vi "Datalogger.vi"   [LabVIEW 2015]
uses:
  DAQ/Controls/Channel Configuration.ctl
  CAN Communication/Oil/Typedefs/Session Handle.ctl
  CAN Communication/Oil/Oil.lvclass
  Common/Buffers/Snapshot/Typedefs/Session Handle.ctl
  Common/Buffers/Snapshot/Snapshot.lvclass
  Common/Circular Error Log/Typedefs/Session Handle.ctl
  Common/Circular Error Log/Circular Error Log.lvclass
  Common/State Machine/State Machine.lvlib
panel:
  # "Datalogger"
types:
  T1 = typedef "Channel Configuration.ctl" = cluster{"Index":u16, "Name":string, "Units":string, "Gain":dbl, "Offset":dbl, "Source":string}
  T2 = typedef "Oil.lvclass/Session Handle.ctl" = refnum<data-value>
  T3 = typedef "Snapshot.lvclass/Session Handle.ctl" = refnum<data-value>
  T4 = typedef "Circular Error Log.lvclass/Session Handle.ctl" = refnum<data-value>
  T5 = cluster{"State":refnum<queue>, "Channels":T1[], "Oil":T2, "Snapshot":T3, "Log Reference":refnum<file>, "LogData":refnum<queue>, "Error":T4, "Log Folder":path}
  T6 = cluster{"Averaged Values":dbl[], "seconds since 1Jan1904":timestamp}
  T7 = enum16{"open", "replace", "create", "open or create", "replace or create", "replace or create with confirmation"}
  T8 = cluster{"Test Name":string, "Test Start":timestamp}
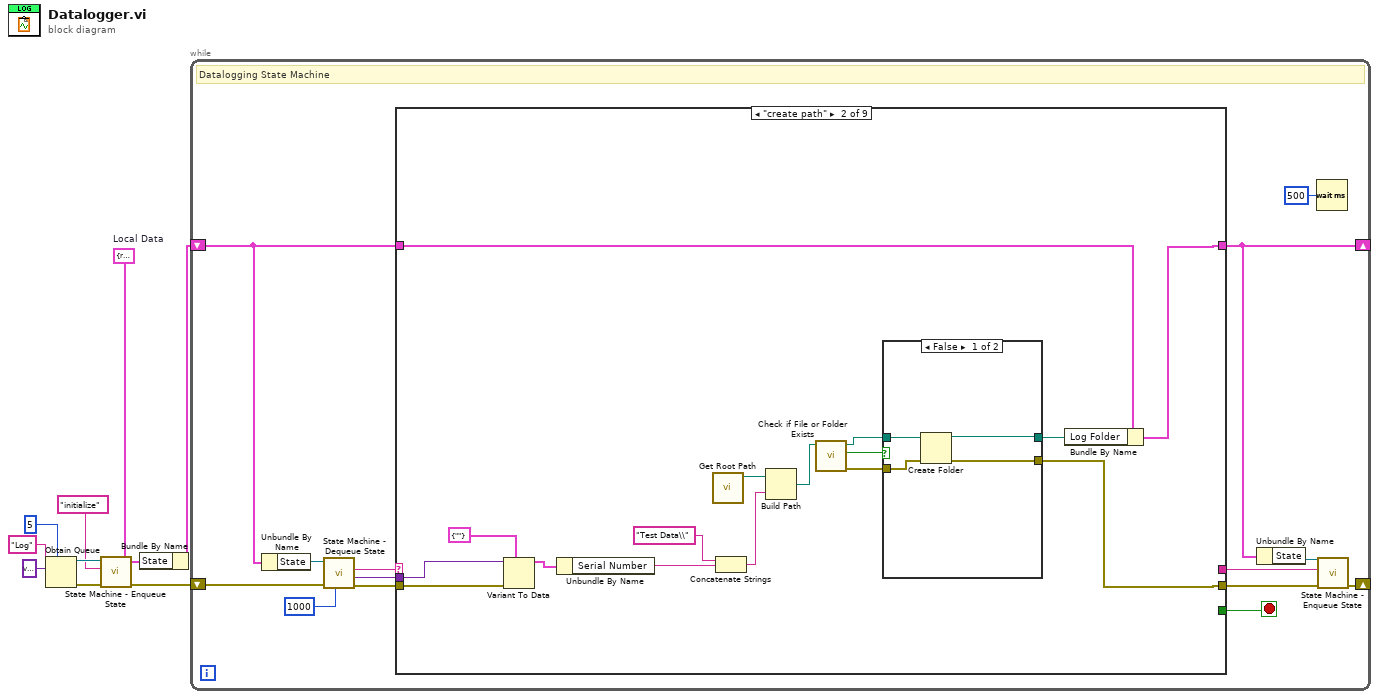
[diagram p0: block diagram]
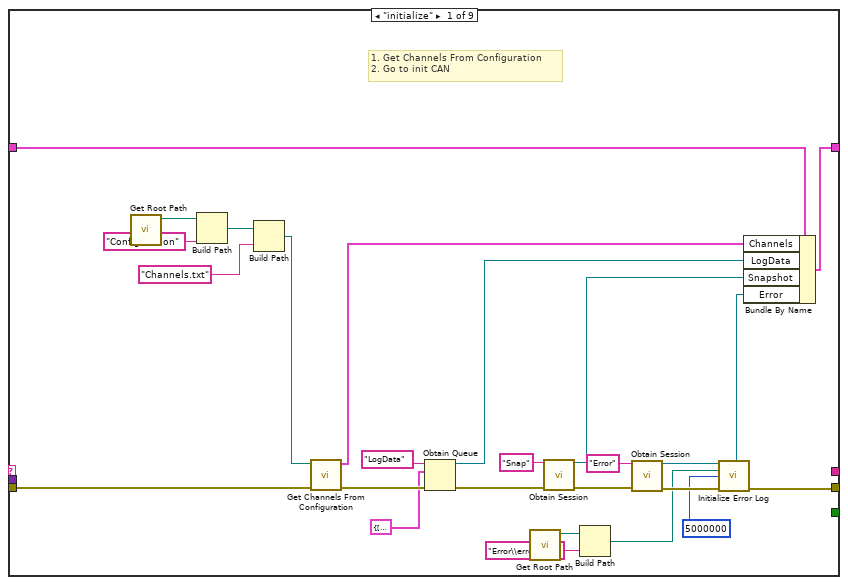
[diagram p2: hidden frame]
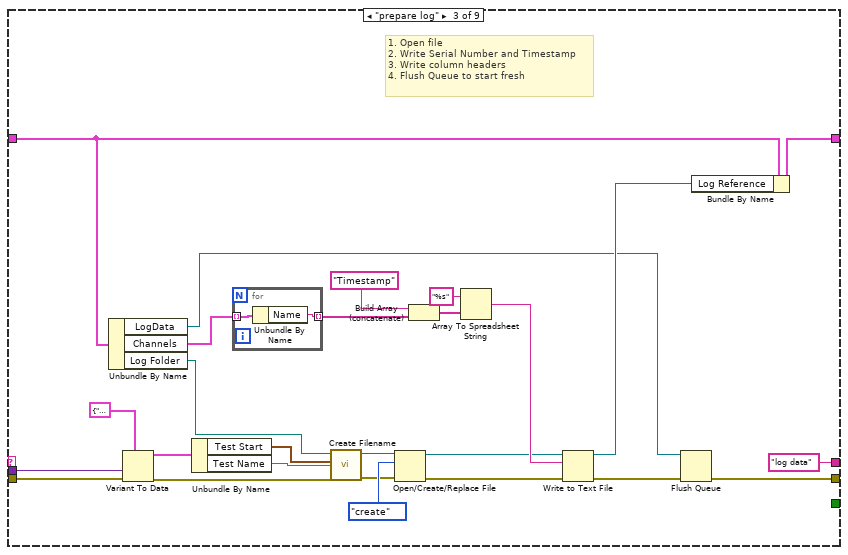
[diagram p4: hidden frame]
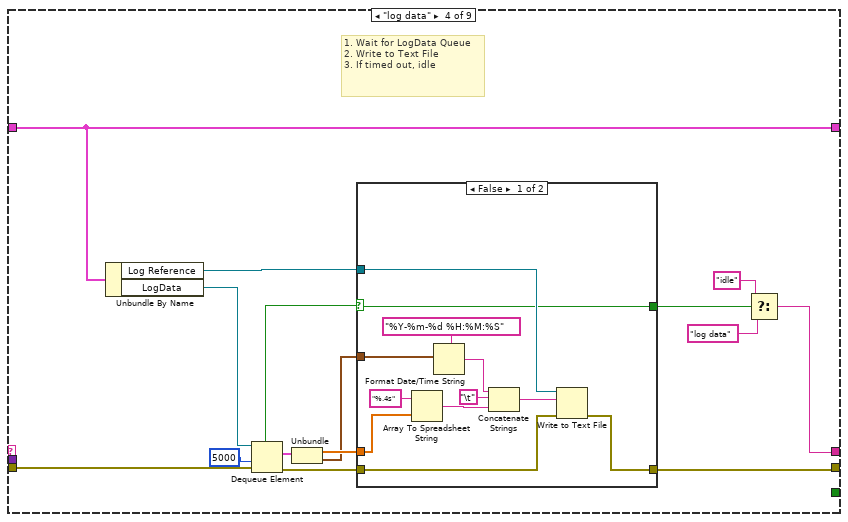
[diagram p5: hidden frame]
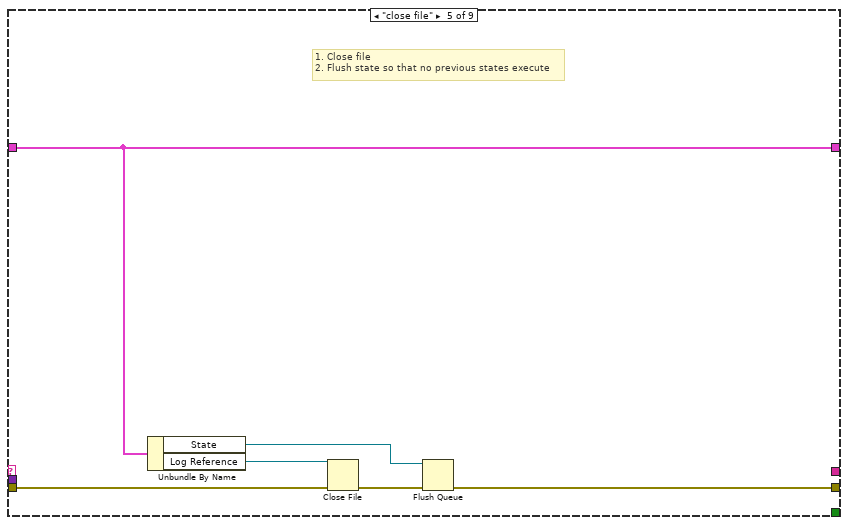
[diagram p7: hidden frame]
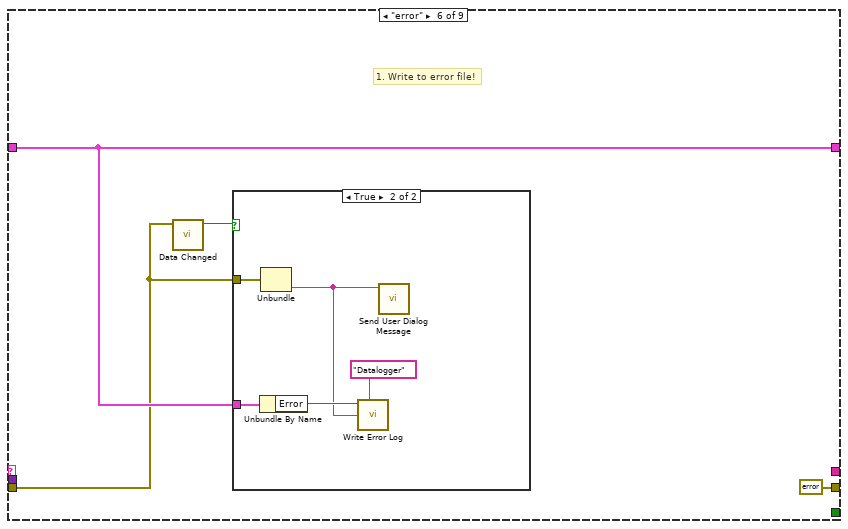
[diagram p8: hidden frame]
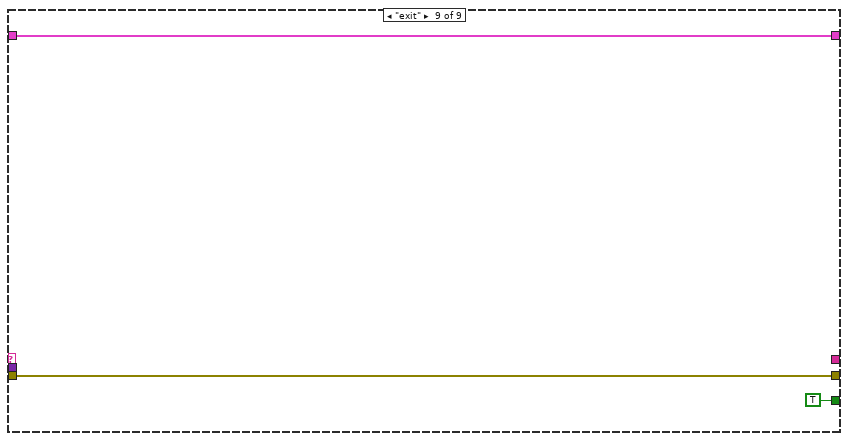
[diagram p12: hidden frame]
diagram:
  w3 = T5 {"State"=refnum, "Channels"=[], "Oil"=refnum, "Snapshot"=refnum, "Log Reference"=refnum, "LogData"=refnum, "Error"=refnum, "Log Folder"=path ""}  # Local Data
  n1 = Obtain Queue(max queue size (-1, unlimited)=5, name (unnamed)="Log", element data type=variant) -> (queue out=w6:refnum<queue>, error out=w7:errorcluster)  [unwired: 2 in, 1 out]
  n2 = call "State Machine - Enqueue State.vi"("error in (no error)"=w7, "State"="initialize", "Queue In"=w6) -> ("error out"=w4:errorcluster, "Queue Out"=w2:refnum<queue>)  [unwired: 7 in]
  n3 = Bundle By Name(cluster=w3, "State"=w2) -> (w1:T5)
  n4 = while "Main State Machine" {
    shift-right: [w21] -> _
    shift-left: w4 -> [w24]
    shift-right: [w12] -> _
    shift-left: w1 -> [w15]
    stop <- w17 stop-if-true
    # "Datalogging State Machine"
    n5 = Unbundle By Name(w15) -> ("State"=w14:refnum<queue>)
    n6 = call "State Machine - Dequeue State.vi"("Timeout"=1000, "error in (no error)"=w24, "Queue In"=w14) -> ("error out"=w23:errorcluster, "Data"=w11:variant, "State"=w22:string)  [unwired: 4 in, 2 out]
    n7 = case shown="\"create path\"" w22 {
      tunnel: w23 -> [w47 w65 w98 w110 w133 w137 w146 w148 w151]
      tunnel: [w30 w51 w78 w105 w130 errorcluster {"status"=FALSE, "code"=0, "source"=""} ("error out") w146 w148 w151] -> w20
      tunnel: [_ _ "log data" ("State") w113 _ _ _ _ _] -> w19
      tunnel: [_ _ _ _ _ _ _ _ TRUE] -> w17
      tunnel: w15 -> [w45 w54 w90 w115 w135 w138 w145 w147 w149]
      tunnel: [w44 w53 w89 w115 w135 w138 w145 w147 w149] -> w12
      tunnel: w11 -> [_ w64 w97 _ _ _ _ _ _]
      frame "initialize" {
        # "1. Get Channels From Configuration\n2. Go to init CAN"
        n8 = call "Get Root Path.vi"() -> ("Root Path"=w28:path)  [unwired: 11 in]
        n9 = Build Path(base path=w28, name or relative path="Configuration") -> (appended path=w49:path)
        n10 = Build Path(base path=w49, name or relative path="Channels.txt") -> (appended path=w46:path)
        n11 = call "Get Channels From Configuration.vi"("error in (no error)"=w47, "Path"=w46) -> ("error out"=w42:errorcluster, "Channels"=w43:T1[])  [unwired: 8 in]
        n12 = Obtain Queue(name (unnamed)="LogData", element data type=T6 {"Averaged Values"=[], "seconds since 1Jan1904"=timestamp(0 s since 1904-01-01)} ("output cluster"), error in (no error)=w42) -> (queue out=w40:refnum<queue>, error out=w39:errorcluster)  [unwired: 2 in, 1 out]
        n13 = call "Get Root Path.vi"() -> ("Root Path"=w27:path)  [unwired: 11 in]
        n14 = call "Obtain Session.vi"("Session  Name ()"="Snap", "error in (no error)"=w39) -> ("Session Handle"=w37:T3, "error out"=w31:errorcluster)  [unwired: 12 in]
        n15 = Build Path(base path=w27, name or relative path="Error\\error.txt") -> (appended path=w25:path)
        n16 = call "Obtain Session.vi"("Session  Name ()"="Error", "error in (no error)"=w31) -> ("Session Handle"=w33:T4, "error out"=w34:errorcluster)  [unwired: 12 in]
        n17 = call "Initialize Error Log.vi"("Session Handle in"=w33, "Error Path"=w25, "Max File Size"=i64 5000000, "error in (no error)"=w34) -> ("Session Handle out"=w29:T4, "error out"=w30:errorcluster)  [unwired: 10 in]
        n18 = Bundle By Name(cluster=w45, "Channels"=w43, "LogData"=w40, "Snapshot"=w37, "Error"=w29) -> (w44:T5)
      }
      frame "create path" {
        n19 = Variant To Data(error in=w65, type=cluster{"Serial Number":string} {"Serial Number"=""}, Variant=w64) -> (data=w63:cluster{"Serial Number":string})  [unwired: 1 out]
        n20 = Unbundle By Name(w63) -> ("Serial Number"=w61:string)
        n21 = call "Get Root Path.vi"() -> ("Root Path"=w62:path)  [unwired: 11 in]
        n22 = Concatenate Strings("Test Data\\" ("string"), w61) -> (w59:string)
        n23 = Build Path(base path=w62, name or relative path=w59) -> (appended path=w58:path)
        n24 = call <vilib>:"Check if File or Folder Exists.vi"("path"=w58) -> ("error out"=w55:errorcluster, "file or folder exists?"=w57:bool, "dup path"=w56:path)  [unwired: 8 in]
        n25 = case shown="False" w57 {
          tunnel: [w68 w72] -> w52
          tunnel: w56 -> [w70 w72]
          tunnel: w55 -> [w69 w71]
          tunnel: [w67 w71] -> w51
          frame False {
            n26 = Create Folder(path (use dialog)=w70, error in=w69) -> (created path=w68:path, error out=w67:errorcluster)  [unwired: 1 in, 1 out]
          }
          frame True {
          }
        }
        n27 = Bundle By Name(cluster=w54, "Log Folder"=w52) -> (w53:T5)
      }
      frame "prepare log" {
        # "1. Open file\n2. Write Serial Number and Timestamp\n3. Write column headers\n4. Flush Queue to start fresh"
        n28 = Unbundle By Name(w90) -> ("LogData"=w79:refnum<queue>, "Channels"=w88:T1[], "Log Folder"=w73:path)
        n29 = Variant To Data(error in=w98, type=T8 {"Test Name"="", "Test Start"=timestamp(0 s since 1904-01-01)}, Variant=w97) -> (data=w95:T8, error out=w75:errorcluster)
        n30 = Unbundle By Name(w95) -> ("Test Start"=w94:timestamp, "Test Name"=w93:string)
        n31 = for {
          tunnel: w88 -> [w100] mode=indexing
          tunnel: [w99] -> w87 mode=indexing
          n32 = Unbundle By Name(w100) -> ("Name"=w99:string)
        }
        n33 = call "Create Filename.vi"("error in (no error)"=w75, "Test Name"=w93, "Test Start"=w94, "Data Folder"=w73) -> ("error out"=w74:errorcluster, "appended path out"=w92:path)  [unwired: 6 in]
        n34 = Open/Create/Replace File(file path (use dialog)=w92, error in=w74, operation (0:open)=T7."create") -> (refnum out=w81:refnum<file>, error out=w83:errorcluster)  [unwired: 3 in, 1 out]
        n35 = Build Array (concatenate)("Timestamp" ("Name"), w87) -> (w85:string[])
        n36 = Array To Spreadsheet String(array=w85, 3:"%s" ("format string")) -> (spreadsheet string=w82:string)  [unwired: 1 in]
        n37 = Write to Text File(file (use dialog)=w81, text=w82, error in=w83) -> (refnum out=w80:refnum<file>, error out=w77:errorcluster)  [unwired: 1 in, 1 out]
        n38 = Flush Queue(queue=w79, error in (no error)=w77) -> (error out=w78:errorcluster)  [unwired: 2 out]
        n39 = Bundle By Name(cluster=w90, "Log Reference"=w80) -> (w89:T5)
      }
      frame "log data" {
        # "1. Wait for LogData Queue\n2. Write to Text File\n3. If timed out, idle"
        n40 = Unbundle By Name(w115) -> ("Log Reference"=w106:refnum<file>, "LogData"=w114:refnum<queue>)
        n41 = Dequeue Element(queue=w114, timeout in ms (-1)=5000, error in (no error)=w110) -> (element=w102:T6, timed out?=w107:bool, error out=w108:errorcluster)  [unwired: 1 out]
        n42 = Unbundle(w102) -> ("Averaged Values"=w103:dbl[], "seconds since 1Jan1904"=w101:timestamp)
        n43 = case shown="False" w107 {
          selector: w107 -> [w122 w128]
          tunnel: w108 -> [w125 w129]
          tunnel: w103 -> [w127 _]
          tunnel: w106 -> [w124 _]
          tunnel: [w123 w129] -> w105
          tunnel: [w122 w128] -> w104
          tunnel: w101 -> [w116 _]
          frame False {
            n44 = Array To Spreadsheet String(array=w127, 3:"%.4s" ("format string")) -> (spreadsheet string=w118:string)  [unwired: 1 in]
            n45 = Format Date/Time String(time format string (%c)="%Y-%m-%d %H:%M:%S", seconds (now)=w116) -> (date/time string=w120:string)  [unwired: 1 in]
            n46 = Concatenate Strings(w120, "\t", w118) -> (w117:string)
            n47 = Write to Text File(file (use dialog)=w124, text=w117, error in=w125) -> (error out=w123:errorcluster)  [unwired: 1 in, 2 out]
          }
          frame True {
          }
        }
        n48 = Select(t="idle" ("State"), s=w104, f="log data" ("State")) -> (s? t:f=w113:string)
      }
      frame "close file" {
        # "1. Close file\n2. Flush state so that no previous states execute"
        n49 = Unbundle By Name(w135) -> ("State"=w131:refnum<queue>, "Log Reference"=w134:refnum<file>)
        n50 = Close File(refnum=w134, error in=w133) -> (error out=w132:errorcluster)  [unwired: 1 out]
        n51 = Flush Queue(queue=w131, error in (no error)=w132) -> (error out=w130:errorcluster)  [unwired: 2 out]
      }
      frame "error" {
        # "1. Write to error file!"
        n52 = call "Data Changed.vi"("Data"=w137) -> ("Changed?"=w136:bool)  [unwired: 10 in]
        n53 = case shown="True" w136 {
          tunnel: w138 -> [_ w142]
          tunnel: w137 -> [_ w141]
          frame False {
          }
          frame True {
            n54 = Unbundle By Name(w142) -> ("Error"=w144:T4)
            n55 = Unbundle(w141) -> ("source"=w140:string)  [unwired: 2 out]
            n56 = call "Write Error Log.vi"("Session Handle in"=w144, "Process Name"="Datalogger", "Data"=w140) -> ()  [unwired: 11 in, 2 out]
            n57 = call "Send User Dialog Message.vi"("Error String"=w140) -> ()  [unwired: 10 in, 1 out]
          }
        }
      }
      frame Default {
      }
      frame "idle" {
      }
      frame "exit" {
      }
    }
    n58 = Unbundle By Name(w12) -> ("State"=w13:refnum<queue>)
    n59 = Wait (ms)(milliseconds to wait=u32 500) -> ()  [unwired: 1 out]
    n60 = call "State Machine - Enqueue State.vi"("error in (no error)"=w20, "State"=w19, "Queue In"=w13) -> ("error out"=w21:errorcluster)  [unwired: 7 in, 1 out]
  }
